vi "Get Port.vi"(11 "Request in":refnum<class "Request.lvclass">) -> (2 "Port":u16)   [LabVIEW 2020, in "OAuth2.lvlib" / "Request.lvclass"]
uses:
  Request.lvclass
  lv-stream/stream/URI/URI.lvclass
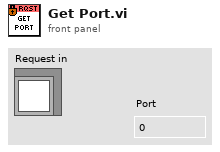
[diagram p1: front panel]
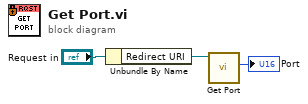
[diagram p0: block diagram]
diagram:
  n1 = Unbundle By Name("Request in") -> ("Redirect URI"=w2:refnum<class "URI.lvclass">)
  n2 = call "Get Port.vi"("URI in"=w2) -> ("Port"=→"Port":u16)  [unwired: 8 in, 2 out]
